vi "Update Measurement Table.vi"(8 "error in (no error)":errorcluster, 11 "AnalogInput in":refnum<class "AnalogInput.lvclass">) -> (0 "error out":errorcluster, 3 "AnalogInput out":refnum<class "AnalogInput.lvclass">)   [LabVIEW 2019, in "AnalogInput.lvlib" / "AnalogInput.lvclass"]
uses:
  Library/AnalogInput.lvclass
  C:/Users/Public/Documents/Development/builds/Instruments/Instruments.lvlibp/Library/Instruments.lvclass
  Library/AnalogInput.lvclass/AnalogInput.ctl
  builds/Instruments/Instruments.lvlibp/Accessors/Read Measured.vi
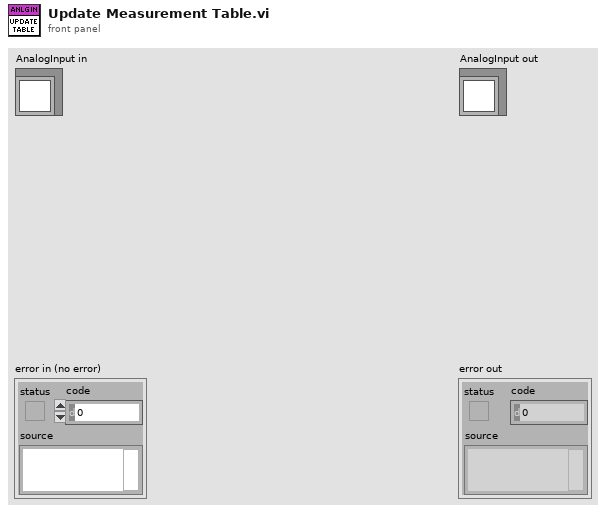
[diagram p1: front panel]
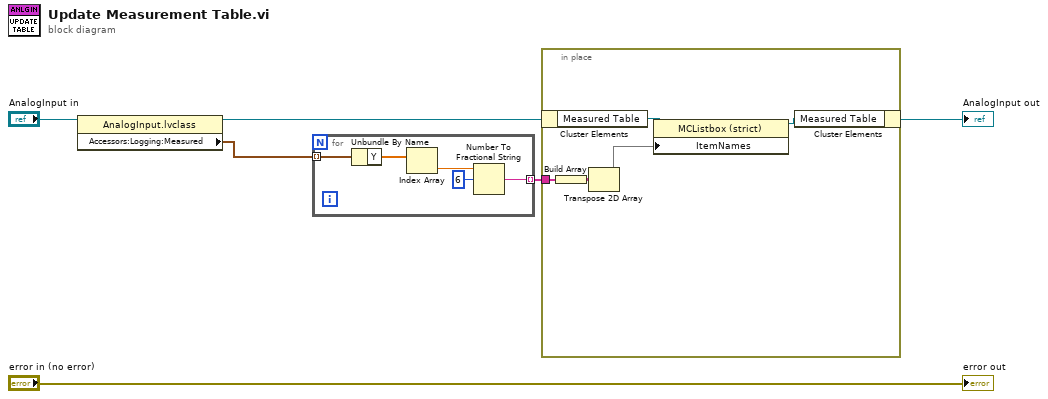
[diagram p0: block diagram]
diagram:
  n1 = property class="AnalogInput.lvclass"(reference="AnalogInput in") -> (reference out=w4:refnum<class "AnalogInput.lvclass">, "Accessors:Logging:Measured"=w5:waveform(dbl)[])  [unwired: 1 in, 1 out]
  n2 = for {
    tunnel: w5 -> [w11] mode=indexing
    tunnel: [w7] -> w2 mode=indexing
    n3 = Unbundle By Name(w11) -> ("Y"=w10:dbl[])
    n4 = Index Array(array=w10) -> (element=w9:dbl)  [unwired: 1 in]
    n5 = Number To Fractional String(number=w9, width (-)=i16 6) -> (F-format string=w7:string)  [unwired: 2 in]
  }
  n6 = in-place {
    in-place-border: w2 -> [w14]
    n7 = in-place-cluster #1(w4) -> ("Measured Table"=w16:refnum<vi>)
    n8 = Build Array(w14) -> (w13:string[][])
    n9 = Transpose 2D Array(2D array=w13) -> (transposed array=w12:string[][])
    n10 = property class="MCListbox (strict)"(reference=w16, "ItemNames"=w12) -> (reference out=w15:refnum<vi>)  [unwired: 1 in, 1 out]
    n11 = in-place-cluster #1("Measured Table"=w15) -> (→"AnalogInput out":refnum<class "AnalogInput.lvclass">)
  }
  "error out" <- "error in (no error)"
